vi "Solution part 1.vi"(11 "data?":bool) -> (3 "result":u64)   [LabVIEW 2020]
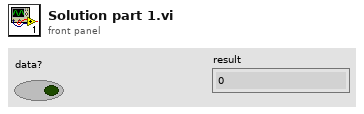
[diagram p1: front panel]
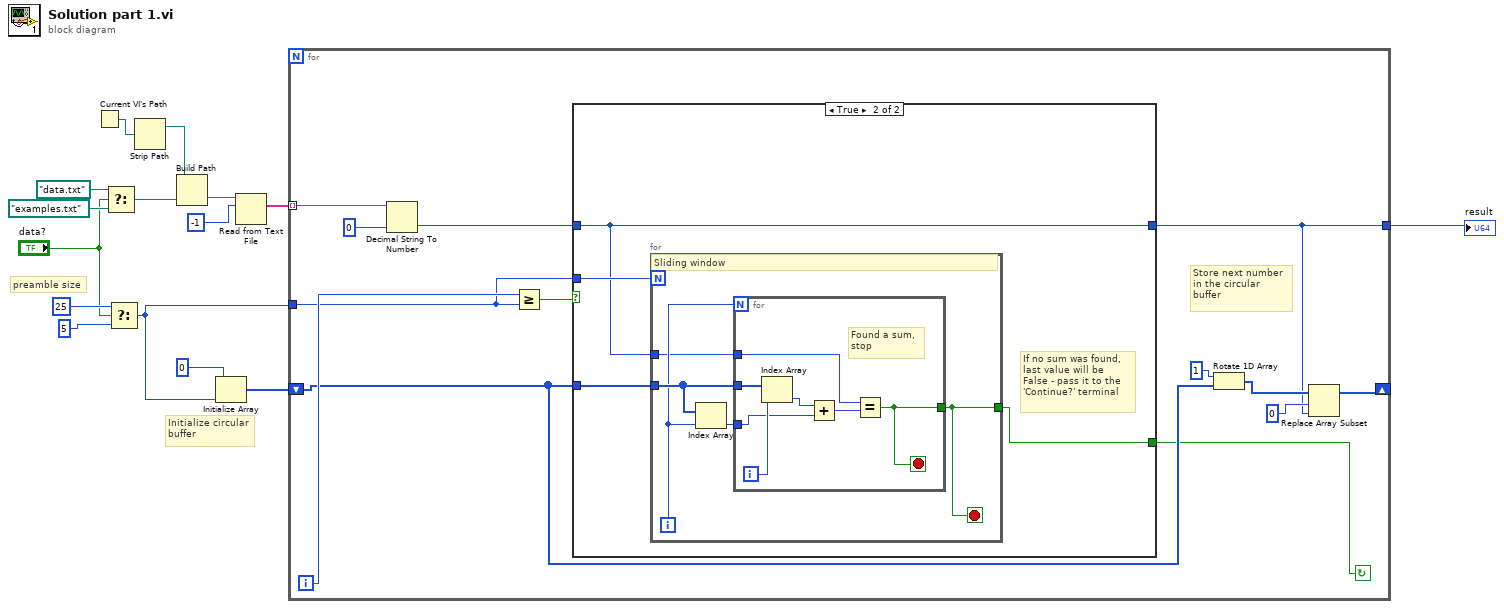
[diagram p0: block diagram]
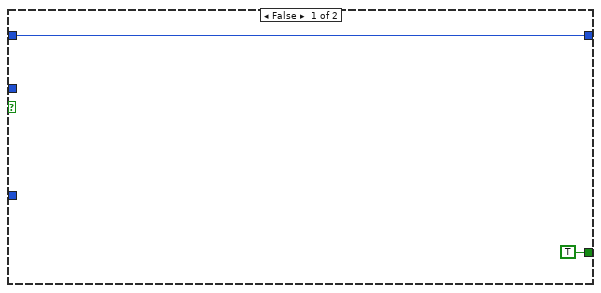
[diagram p2: hidden frame]
diagram:
  # "Initialize circular\nbuffer"
  # "preamble size"
  n1 = Current VI's Path() -> (path=w12:path)
  n2 = Select(t=path "data.txt", s="data?", f=path "examples.txt") -> (s? t:f=w13:path)
  n3 = Select(t=25 ("count"), s="data?", f=5 ("count")) -> (s? t:f=w2:i32)
  n4 = Strip Path(path=w12) -> (stripped path=w11:path)  [unwired: 1 out]
  n5 = Build Path(base path=w11, name or relative path=w13) -> (appended path=w10:path)
  n6 = Initialize Array(u64 0 ("count"), w2) -> (w3:u64[])
  n7 = Read from Text File(file (use dialog)=w10, count=-1) -> (text=w8:string[])  [unwired: 2 in, 3 out]
  n8 = for {
    tunnel: w8 -> [w28] mode=indexing
    shift-right: [w20] -> _
    shift-left: w3 -> [w19]
    tunnel: w2 -> [w24]
    tunnel: [w17] -> w1
    i -> [w26]
    stop <- w18 continue-if-true
    # "Store next number\nin the circular\nbuffer"
    n9 = Decimal String To Number(string=w28, default (0L)=u64 0 ("count")) -> (number=w23:u64)  [unwired: 1 in, 1 out]
    n10 = Greater Or Equal?(x=w26, y=w24) -> (x >= y?=w25:bool)
    n11 = case shown="True" w25 {
      tunnel: w19 -> [_ w32]
      tunnel: w24 -> [_ w34]
      tunnel: w23 -> [w30 w33]
      tunnel: [w30 w33] -> w17
      tunnel: [TRUE w31] -> w18
      frame False {
      }
      frame True {
        # "If no sum was found,\nlast value will be \nFalse - pass it to the\n'Continue?' terminal"
        n12 = for {
          N: w34 -> [_]
          tunnel: w33 -> [w36]
          tunnel: w32 -> [w38]
          tunnel: [w35] -> w31
          i -> [w37]
          stop <- w35 stop-if-true
          # "Sliding window"
          n13 = Index Array(array=w38, index=w37) -> (element=w39:u64)
          n14 = for {
            N: w37 -> [_]
            tunnel: w39 -> [w43]
            tunnel: w38 -> [w46]
            tunnel: w36 -> [w41]
            tunnel: [w40] -> w35
            i -> [w45]
            stop <- w40 stop-if-true
            # "Found a sum,\nstop"
            n15 = Index Array(array=w46, index=w45) -> (element=w44:u64)
            n16 = Add(x=w44, y=w43) -> (x+y=w42:u64)
            n17 = Equal?(x=w41, y=w42) -> (x = y?=w40:bool)
          }
        }
      }
    }
    n18 = Rotate 1D Array(1:w19, 2:1 ("n")) -> (0:w21:u64[])
    n19 = Replace Array Subset(array=w21, new element=w17, index=0) -> (w20:u64[])
  }
  "result" <- w1
